vi "ImagerForFlowbit5_led_screenSensor.vi"() -> ()   [LabVIEW 2011]
uses:
  <vilib>/vision/Image Controls.llb/IMAQ Image.ctl
  <vilib>/Platform/TimedLoop/XDataNode/timing_clust.ctl
  <vilib>/Platform/TimedLoop/XDataNode/nitl_modes.ctl
  <vilib>/Platform/TimedLoop/XDataNode/wakeup.ctl
  <vilib>/Utility/config.llb/Read Key (I32).vi
  <vilib>/Analysis/1siggen.llb/Riffle Array (I32).vi
  <vilib>/Platform/TimedLoop/XDataNode/XDataNode.xnode
  <vilib>/Analysis/NI_AALBase.lvlib
  <vilib>/vision/NI_Vision_Development_Module.lvlib
  <vilib>/Platform/TimedLoop/XDataNode/XDNodeRunTimeDep.lvlib
  <vilib>/Utility/config.llb/NI_LVConfig.lvlib
panel:
  out "ScreenSensor":bool
  out "onLineMapOutput":T1[](array[typedef])
  out "Bounds.Right":i16
  out "停止循环":bool
  in  "Stimuli":i64=5
  in  "选项卡控件":enum32{"前面板", "参数设置", "OnLineMap"}(tab)
  in  "shutter":bool
  out "log":string
  out "Stim_ID":i32(listbox)=1
  in  "开始/暂停":bool=TRUE
  in  "停止":bool
  out "重排的 Stim ID":i32[](array[numeric]) caption="重排的{X}"
  out "block":i32
  out "队列中元素数量":i32
  out "Image 2":T1(plugin-control)
  in  "热图":bool
  out "循环持续时间":i64
  out "Recording":bool
  out "grabLoop":i32
  out "writeing data":bool
  out "address":i16=888 caption="地址" format="%.0x"
  in  "SaveParameter":bool
  in  "Pra_binType":enum16{"Extract", "Resample"}(ring)
  in  "Pra_FramesPerStim":i64=16
  in  "Pra_Blk目录":path=path "D:/Expt/test"
  in  "Pra_文件名":string="G4_E02"
  in  "Pra_TimeForPrepare(ms)":u32=1000
  in  "Pra_stim ID":u8[](array[numeric])=[0, 2, 4, 6, 8]
  in  "Pra_blk总数":i32=500
  in  "Pra_stim protocol":T2(array[ring])=[enum."prep stim", enum."wait respirator", enum."show stim", enum."recording data", enum."Blank stim", enum."writing data", enum."ISI"]
  in  "Pra_blank stim":u8
  in  "Pra_wait（ms）":u32=10
  in  "Pra_ISI（ms）":u32=8000
  in  "Pra_FrameBin":i32=25
  in  "Pra_datatype":u16(ring)=13 items=["U8"=11, "I16"=12, "U32"=13, "SGL"=14]
  in  "FrameWidth":i64=704
  in  "FrameHeight":i64=576
  in  "LoadParameter":bool
  in  "Pra_bin":enum16{"1*1", "2*2"}(ring)
  in  "Pra_DR/R parameter":T3={"frame_zero_0"=0, "frame_zero_1"=1, "frame_0"=3, "frame_1"=15}
  in  "Pra_OnlineMap":cluster{"数组 1":i32[], "数组 2":i32[]}[](array[cluster])=[{"数组 1"=[2], "数组 2"=[6]}, {"数组 1"=[4], "数组 2"=[8]}, {"数组 1"=[2, 6], "数组 2"=[4, 8]}, {"数组 1"=[2, 4, 6, 8], "数组 2"=[0]}, {"数组 1"=[2, 4], "数组 2"=[6, 8]}]
  in  "Pra_clip ratio":dbl=2.0 min=0.0001 step=0.1
  # "-"
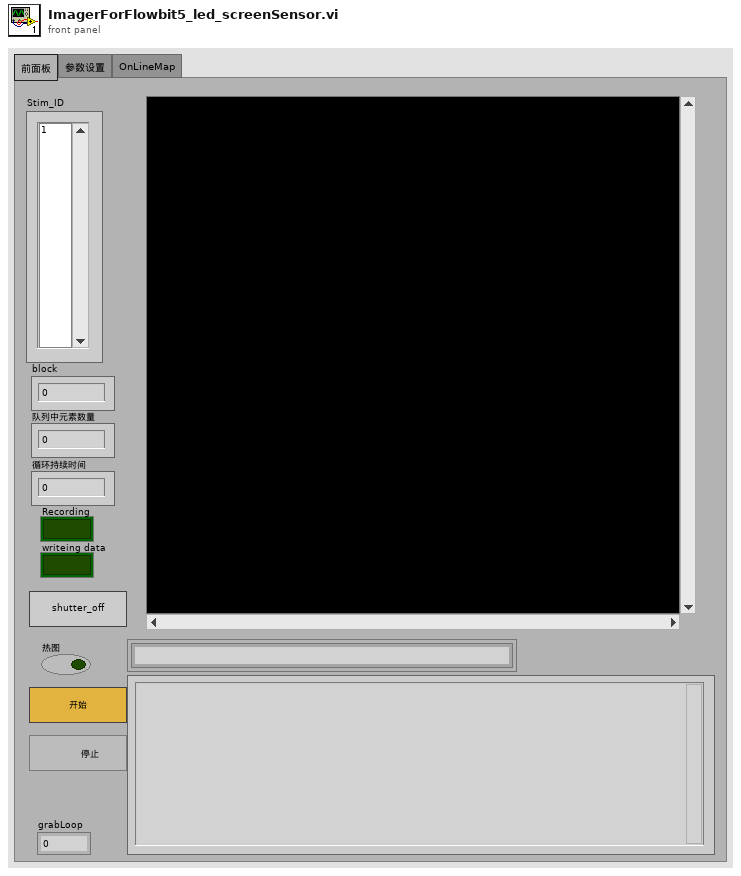
[diagram p1: front panel]
types:
  T1 = typedef "IMAQ Image.ctl" = refnum<image>
  T2 = enum16{"wait", "prep stim", "show stim", "wait respirator", "recording data", "Blank stim", "wait heart", "ISI", "DR/R", "wait calibrate", "openLightShutter", "closeLightShutter", "writing data"}[]
  T3 = cluster{"frame_zero_0":i32, "frame_zero_1":i32, "frame_0":i32, "frame_1":i32}
  T4 = typedef "Image Type" = u32
  T5 = enum16{"Disable External Trigger", "Enable External Trigger"}
  T6 = enum32{"Auto Detect", "RoadRunner", "Raven", "R64"}
  T7 = typedef "LVAllMonitorsDisplayTypeDef.ctl" = cluster{"Bounds":cluster{"Left":i16, "Top":i16, "Right":i16, "Bottom":i16}, "Depth":i16}[]
  T8 = cluster{"Bounds":cluster{"Left":i16, "Top":i16, "Right":i16, "Bottom":i16}, "Depth":i16}
  T9 = typedef "NI_LVConfig.lvlib/Config Data RefNum.ctl" = refnum<k1>
  T10 = typedef "XDNodeRunTimeDep.lvlib/timing_clust.ctl" = cluster{"Expected End [f-1]":u64, "Actual End [f-1]":u64, "Finished Late? [f-1]":bool, "Expected End [i-1]":u64, "Actual End [i-1]":u64, "Finished Late? [i-1]":bool, "Expected Start [i]":u64, "Actual Start [i]":u64, "Expected Start [f]":u64, "Actual Start [f]":u64, "Source Name":string, "Structure Name":string, "Period":i64, "Deadline":i64, "Offset":i64, "Start":i64, "Priority":i32, "Timeout":i32, "Mode":T11, "Wakeup Reason":T12, "Error":errorcluster, "Source Type":string, "Secondary Source Type":string, "Global End Time":u64, "Global Start Time":u64, "Frame Duration":u64, "Iteration Duration":u64, "Assigned CPU":i32, "I/O Scan Engine Mode":u32}
  T11 = typedef "XDNodeRunTimeDep.lvlib/nitl_modes.ctl" = enum32{"No Change", "Process missed periods, maintain original phase", "Discard missed periods, maintain original phase", "Process missed periods, ignore original phase", "Discard missed periods, ignore original phase"}
  T12 = typedef "XDNodeRunTimeDep.lvlib/wakeup.ctl" = enum32{"Normal", "Aborted", "Asynchronous wakeup", "Timing source error", "Timed loop error", "Timeout"}
  T13 = enum16{"big-endian, network order", "native, host order", "little-endian"}
  T14 = enum8{"Enabled", "Disabled", "Disabled and Grayed Out"}
  T15 = enum16{"open", "replace", "create", "open or create", "replace or create", "replace or create with confirmation"}
  T16 = cluster{"Browser Size":cluster{"X":i32, "Y":i32}, "Images per Line":i32, "Background Color":u32, "Frame Size":i32, "Frame Style":enum16{"Raised", "Bevelled", "Outline", "Hidden", "Step", "Raised Outline"}}
  T17 = cluster{"Desired Font (Application)":enum16{"User-specified Font", "Application Font", "System Font", "Dialog Font"}, "[User-specified Font]":cluster{"Font Name":string, "Size":i16, "Strikeout?":bool, "Italic?":bool, "Underline?":bool, "Outline?":bool, "Shadow?":bool, "Bold?":bool, "Rotation Angle":dbl}, "Horizontal Alignment":i16, "Vertical Alignment":i16}
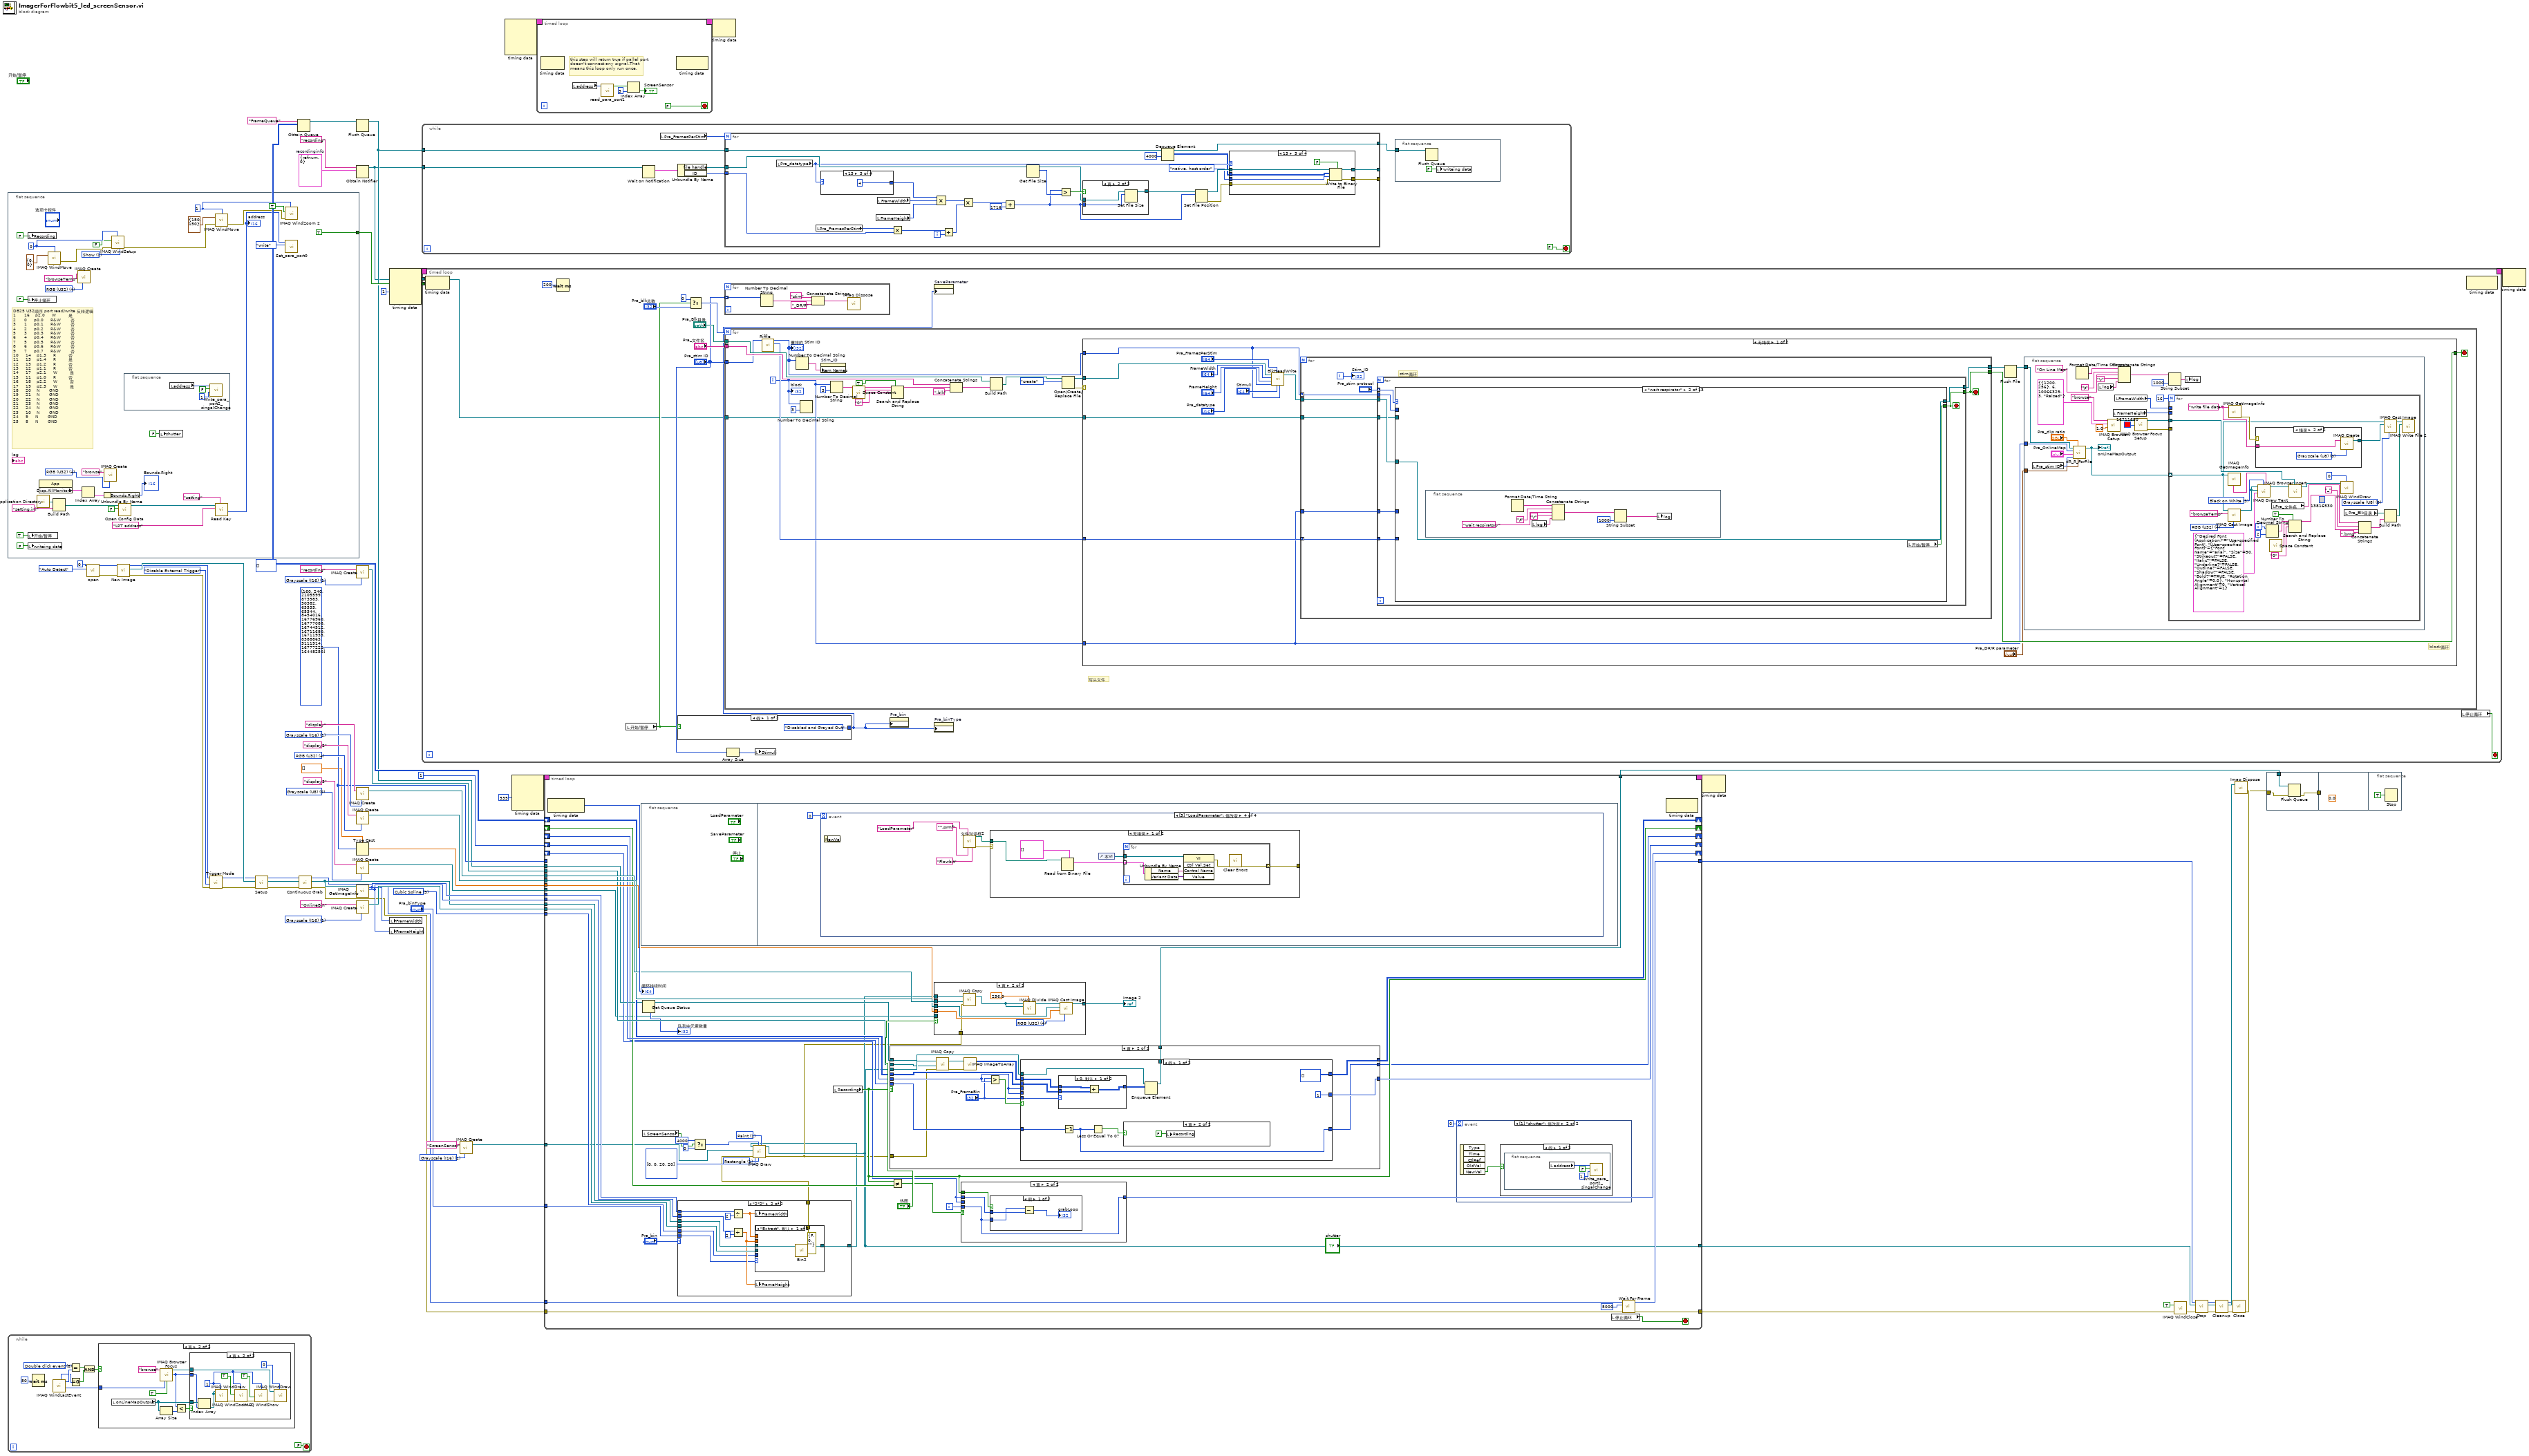
[diagram p0: block diagram]
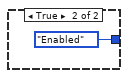
[diagram p2: hidden frame]
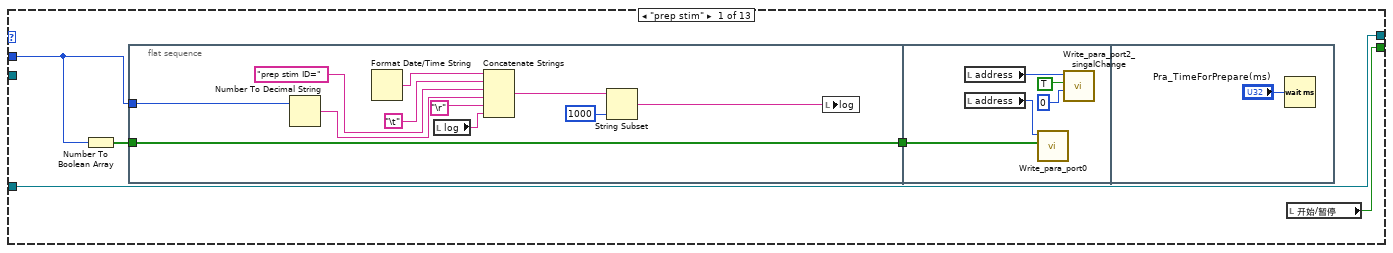
[diagram p4: hidden frame]
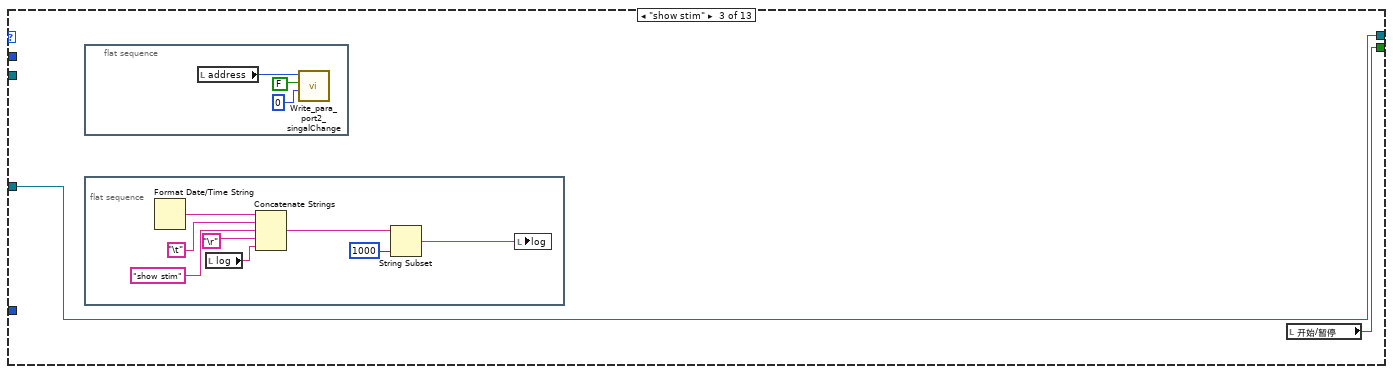
[diagram p5: hidden frame]
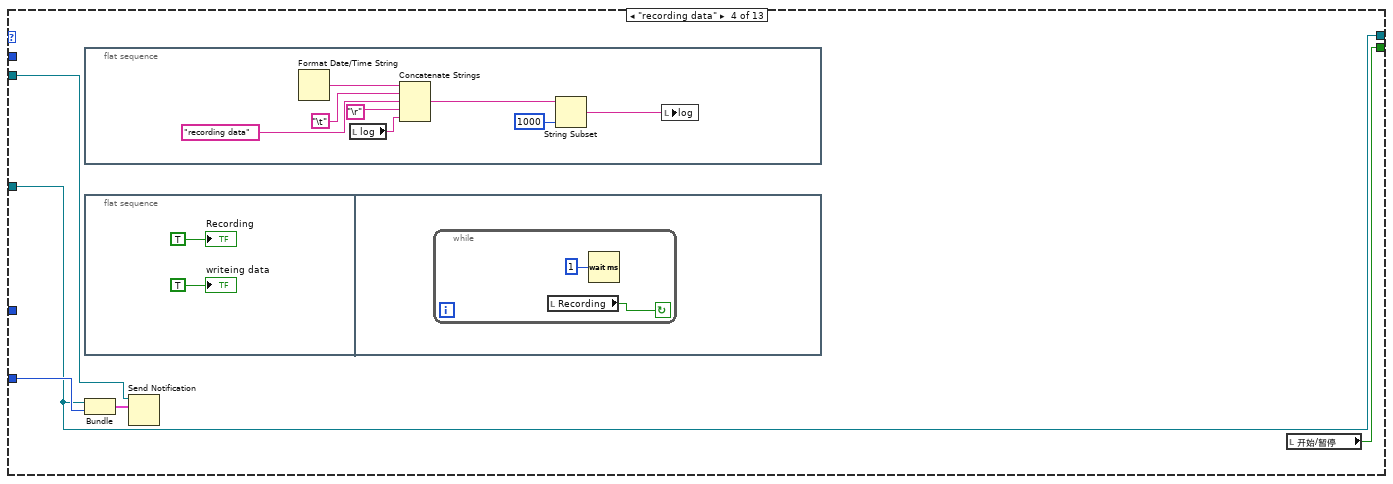
[diagram p6: hidden frame]
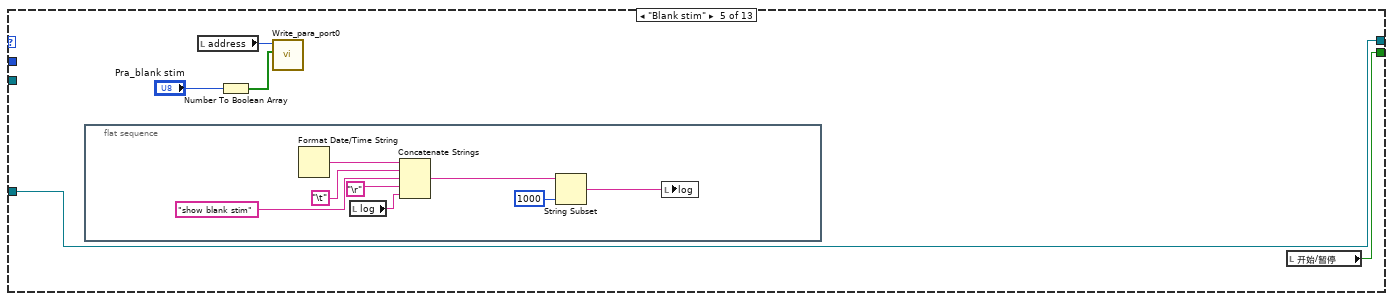
[diagram p7: hidden frame]
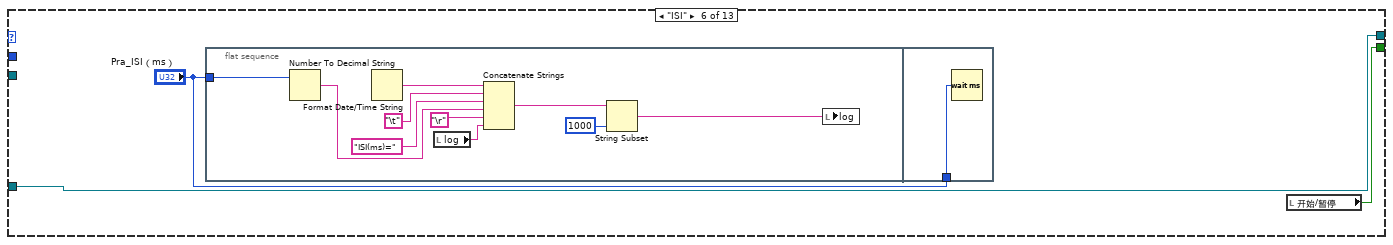
[diagram p8: hidden frame]
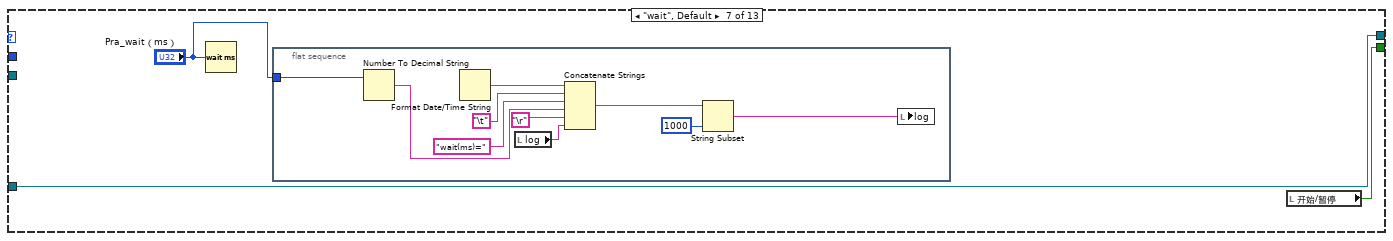
[diagram p9: hidden frame]
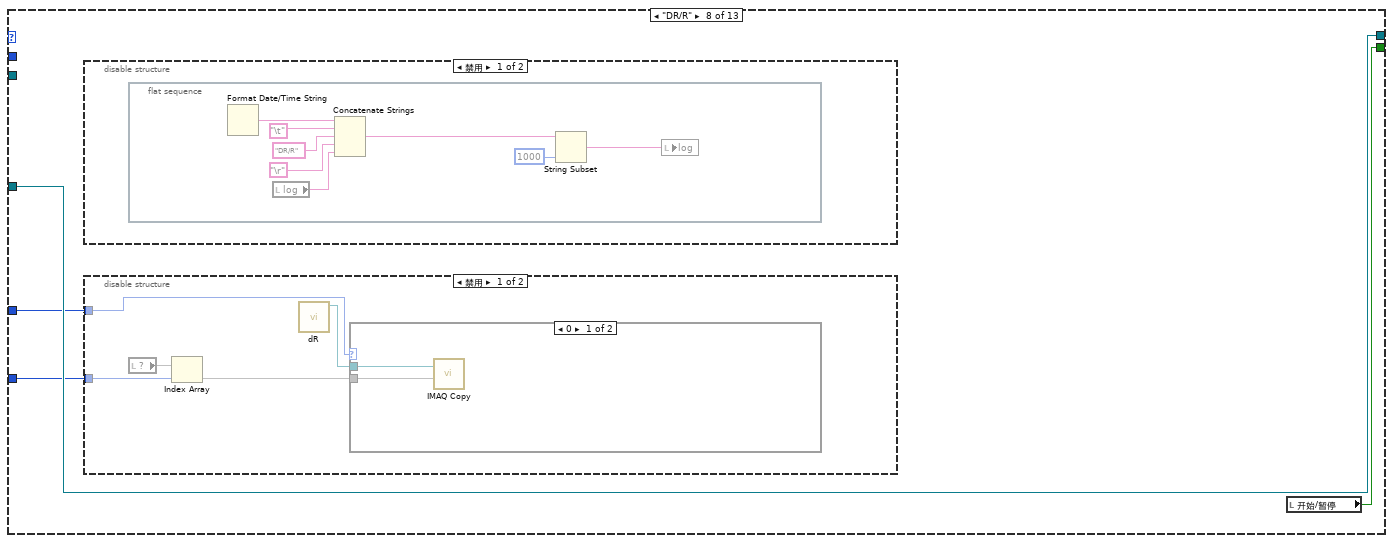
[diagram p10: hidden frame]
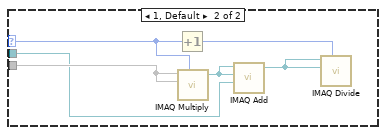
[diagram p12: hidden frame]
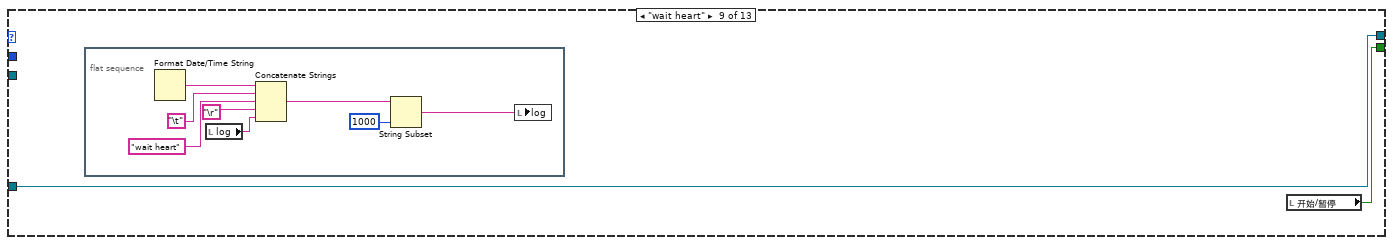
[diagram p14: hidden frame]
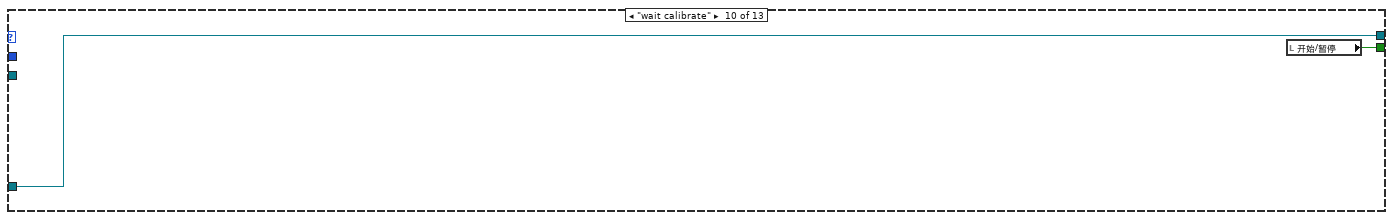
[diagram p15: hidden frame]
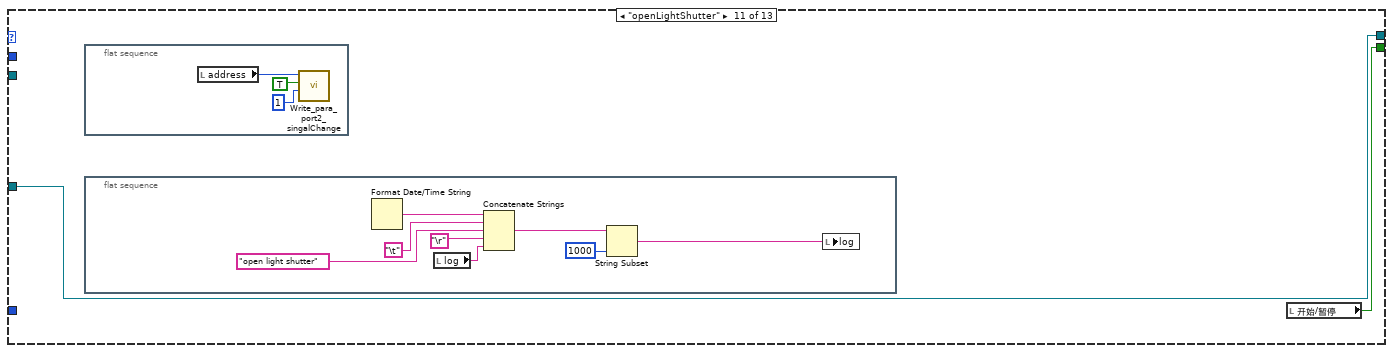
[diagram p16: hidden frame]
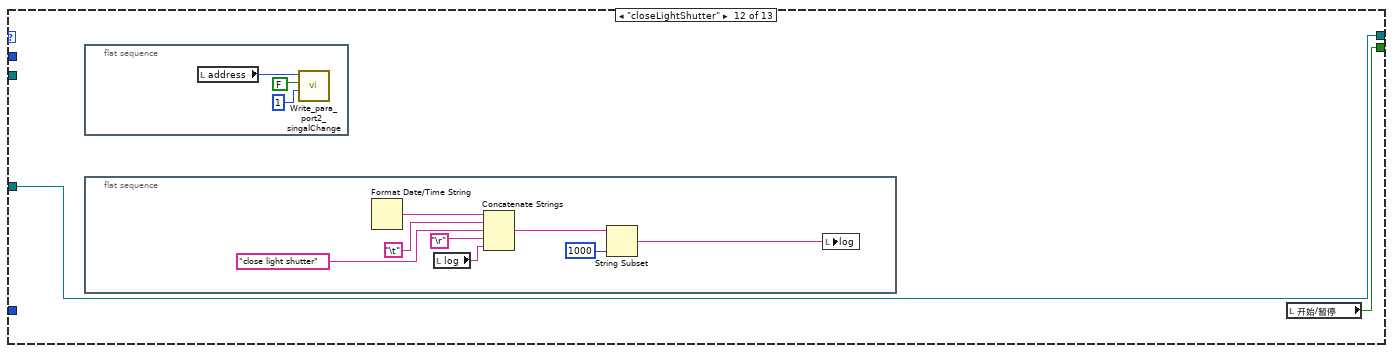
[diagram p17: hidden frame]
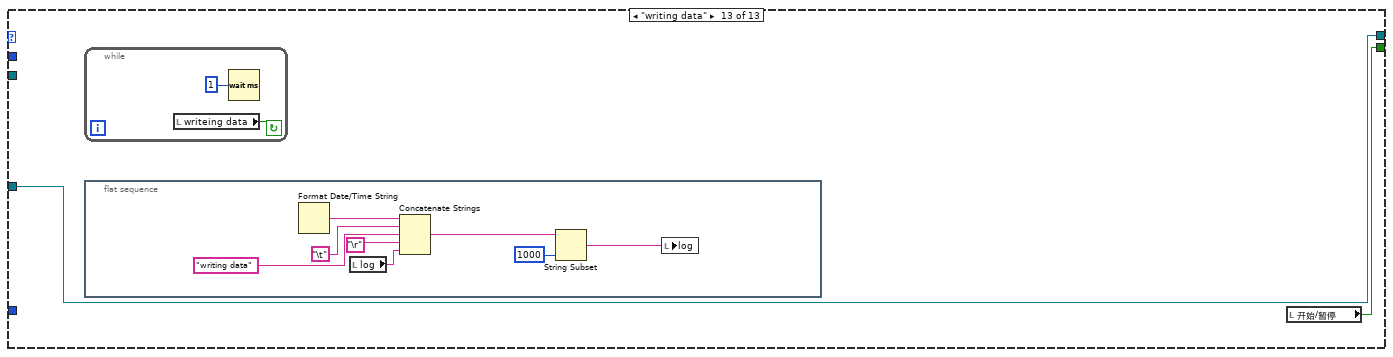
[diagram p18: hidden frame]
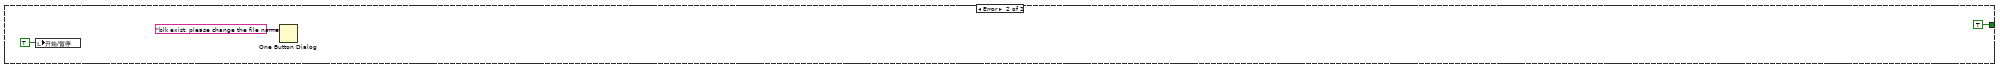
[diagram p19: hidden frame]
diagram:
  w6 = T4 1 items=["Grayscale (U8)", "Grayscale (I16)", "Grayscale (SGL)", "Complex (CSG)", "RGB (U32)", "HSL (U32)", "RGB (U64)", "Grayscale (U16)"] ("Image Type")
  w19 = cluster{"file handle":refnum<file>, "ID":i32} {"file handle"=refnum, "ID"=0}  # recordinginfo
  w24 = T4 0 items=["Grayscale (U8)", "Grayscale (I16)", "Grayscale (SGL)", "Complex (CSG)", "RGB (U32)", "HSL (U32)", "RGB (U64)", "Grayscale (U16)"] ("Image Type")
  w29 = u32 3 items=["Zero Order", "Bi-Linear", "Quadratic", "Cubic Spline"] ("Interpolation Type")
  w31 = T4 1 items=["Grayscale (U8)", "Grayscale (I16)", "Grayscale (SGL)", "Complex (CSG)", "RGB (U32)", "HSL (U32)", "RGB (U64)", "Grayscale (U16)"] ("Image Type")
  w33 = u32[][] []
  w42 = T4 4 items=["Grayscale (U8)", "Grayscale (I16)", "Grayscale (SGL)", "Complex (CSG)", "RGB (U32)", "HSL (U32)", "RGB (U64)", "Grayscale (U16)"] ("Image Type")
  w40 = u32[] [160, 240, 2105599, 873983, 50382, 65535, 65344, 8454016, 16776960, 16777088, 16744512, 16711680, 16711935, 8388863, 5111914, 16777222, 16448250] ("数组")
  w46 = T4 1 items=["Grayscale (U8)", "Grayscale (I16)", "Grayscale (SGL)", "Complex (CSG)", "RGB (U32)", "HSL (U32)", "RGB (U64)", "Grayscale (U16)"] ("Image Type")
  w47 = T4 1 items=["Grayscale (U8)", "Grayscale (I16)", "Grayscale (SGL)", "Complex (CSG)", "RGB (U32)", "HSL (U32)", "RGB (U64)", "Grayscale (U16)"] ("Image Type")
  n1 = flat-sequence {
    tunnel: [TRUE ("Zoom to Fit Mode")] -> w35
    frame #0 {
      w80 = 1 items=["Hide", "Show", "No change"] ("Scrollbars (No change)")
      w77 = 1 ("Window Number (0...15)")
      w81 = 0 ("Window Number (0...15)")
      w86 = T4 4 items=["Grayscale (U8)", "Grayscale (I16)", "Grayscale (SGL)", "Complex (CSG)", "RGB (U32)", "HSL (U32)", "RGB (U64)", "Grayscale (U16)"] ("Image Type")
      w87 = T4 4 items=["Grayscale (U8)", "Grayscale (I16)", "Grayscale (SGL)", "Complex (CSG)", "RGB (U32)", "HSL (U32)", "RGB (U64)", "Grayscale (U16)"] ("Image Type")
      # "DB25\tU32顺序\tport\tread/write\t反转逻辑\n1\t     16\t   p2.0    \tW\t        是\n2\t     0    \tp0.0\t   \tR&W\t      否\n3\t     1\t\t   p0.1\t   \tR&W      \t否\n4\t\t    2\t   \tp0.2   \t\tR&W      \t否\n5\t\t    3\t\t   p0.3   \t\tR&W\t      否\n6\t\t    4\t   \tp0.4   \t\tR&W      \t否\n7\t\t    5\t   \tp0.5   \t\tR&W      \t否\n8\t\t    6\t   \tp0.6\t   \tR&W      \t否\n9\t    \t7\t   \tp0.7\t   \tR&W\t      否\n10\t    14   \tp1.3   \t\tR        \t否\n11\t   \t15   \tp1.4   \t\tR        \t是\n12\t   \t13   \tp1.2\t   \tR        \t否\n13    \t12   \tp1.1\t   \tR        \t否\n14     17   \tp2.1\t   \tW        \t是\n15    \t11   \tp1.0   \t\tR\t        否\n16    \t18   \tp2.2   \t\tW        \t否\n17    \t19\t   p2.3   \t\tW\t        是\n18    \t20   \tN   \t  \tGND\t\n19    \t21   \tN   \t  \tGND\t\n20\t    22\t   N\t  \t  \tGND\t\n21\t    23\t   N  \t  \t\tGND\t\n22\t    24\t   N  \t  \t\tGND\t\n23    \t10   \tN  \t  \t\tGND\t\n24    \t9\t    N  \t  \t\tGND\t\n25\t    8    \tN  \t  \t\tGND"
      n2 = local write "Recording"(FALSE ("Recording")) -> ()
      n3 = local write "停止循环"(FALSE ("开始/暂停")) -> ()
      n4 = local write "开始/暂停"(TRUE ("开始/暂停")) -> ()
      n5 = local write "writeing data"(FALSE ("Recording")) -> ()
      n6 = call <vilib>:"Application Directory.vi"() -> ("Application Directory"=w99:path)
      n7 = property class="App"() -> ("Disp.AllMonitors"=w91:T7)  [unwired: 2 in, 2 out]
      n8 = call "IMAQ WindMove"("Window Number (0...15)"=w81, "Coordinates (screen)"=cluster{"X Position":i32, "Y Position":i32} {"X Position"=0, "Y Position"=0}) -> ("error out"=w82:errorcluster)  [unwired: 3 in, 1 out]
      n9 = Build Path(base path=w99, name or relative path="setting.ini" ("名称或相对路径")) -> (appended path=w97:path)
      n10 = call "IMAQ Create"("Image Name"="browseTemp", "Image Type"=w86) -> ()  [unwired: 3 in, 2 out]
      n11 = Index Array(array=w91) -> (element=w90:T8)  [unwired: 1 in]
      n12 = call "IMAQ Create"("Image Name"="browse", "Image Type"=w87) -> ()  [unwired: 3 in, 2 out]
      n13 = Unbundle By Name(w90) -> ("Bounds.Right"=→"Bounds.Right":i16)
      n14 = call "IMAQ WindSetup"("Scrollbars (No change)"=w80, "Window Number (0...15)"=w81, "error in (no error)"=w82, "Window can close? (Yes)"=FALSE) -> ("error out"=w79:errorcluster)  [unwired: 7 in]
      n15 = call <vilib>:"Open Config Data.vi"("create file if necessary (T)"=FALSE, "configuration file path"=w97) -> ("refnum"=w95:T9)  [unwired: 7 in, 2 out]
      n16 = flat-sequence {
        frame #0 {
          n17 = local read "address"() -> (w106:i16)
          n18 = call "Write_para_port2_singalChange.vi"("索引"=1, "布尔"=FALSE, "address"=w106) -> ()  [unwired: 8 in, 1 out]
        }
      }
      n19 = local write "shutter"(FALSE ("shutter")) -> ()
      n20 = call "IMAQ WindMove"("Window Number (0...15)"=w77, "Coordinates (screen)"=cluster{"X Position":i32, "Y Position":i32} {"X Position"=150, "Y Position"=150}, "error in (no error)"=w79) -> ("error out"=w78:errorcluster)  [unwired: 2 in, 1 out]
      n21 = call-poly <vilib>:"Read Key.vi"("section"="setting", "key"="LPT address", "refnum"=w95) -> ("value"=w92:i32)  [unwired: 5 in, 3 out]
      "address" <- w92
      n22 = call "IMAQ WindZoom 2"("Window Number (0...15)"=w77, "error in (no error)"=w78, "Zoom to Fit? (False)"=TRUE) -> ()  [unwired: 5 in, 4 out]
      n23 = call "Set_para_port0.vi"("R or W"=enum16{"read", "write"}."write", "address"=w92) -> ()  [unwired: 8 in, 2 out]
    }
  }
  n24 = while {
    stop <- FALSE stop-if-true
    w115 = 8 items=["No  event", "Click event", "Draw event", "Move event", "Size event", "Scroll event", "Activate event", "Close event", "Double click event"] ("Event")
    n25 = Wait (ms)(milliseconds to wait=u32 50 ("等待时间（毫秒）")) -> ()  [unwired: 1 out]
    n26 = call "IMAQ WindLastEvent"() -> ("Coordinates"=w109:i32[], "Event"=w114:i32, "Window Number (0...15)"=w113:i32)  [unwired: 6 in, 3 out]
    n27 = Equal?(x=w115, y=w114) -> (x = y?=w112:bool)
    n28 = Equal To 0?(x=w113) -> (x = 0?=w111:bool)
    n29 = And(x=w112, y=w111) -> (x .and. y?=w110:bool)
    n30 = case shown="真" w110 {
      tunnel: w109 -> [_ w125]
      frame False {
      }
      frame True {
        n31 = local read "onLineMapOutput"() -> (w121:T1[])
        n32 = call "IMAQ Browser Focus"("Image Browser In"="browse" ("Image Name"), "Pixel Position"=w125, "Get/Set (Set)"=TRUE) -> ("Image Browser Out"=w119:T1, "Index Out"=w120:i32)  [unwired: 5 in, 6 out]
        n33 = Array Size(array=w121) -> (size(s)=w123:i32)
        n34 = Less?(x=w120, y=w123) -> (x < y?=w122:bool)
        n35 = case shown="真" w122 {
          tunnel: w121 -> [_ w136]
          tunnel: w120 -> [_ w135]
          tunnel: w119 -> [_ w133]
          frame False {
          }
          frame True {
            w127 = 1 ("Window Number (0...15)")
            n36 = Index Array(array=w136, index=w135) -> (element=w134:T1)
            n37 = call "IMAQ WindDraw"("Window Number (0...15)"=w127, "Title"=w134, "Image"=w134) -> ("error out"=w130:errorcluster)  [unwired: 7 in, 1 out]
            n38 = call "IMAQ WindZoom 2"("Window Number (0...15)"=w127, "error in (no error)"=w130, "Zoom to Fit? (False)"=TRUE) -> ("error out"=w129:errorcluster)  [unwired: 5 in, 3 out]
            n39 = call "IMAQ WindShow"("error in (no error)"=w129, "Bring To Front? (N)"=TRUE, "Window Number (0...15)"=w127) -> ("error out"=w128:errorcluster)  [unwired: 3 in, 2 out]
            n40 = call "IMAQ WindDraw"("Window Number (0...15)"=0, "error in (no error)"=w128, "Image"=w133) -> ()  [unwired: 7 in, 2 out]
          }
        }
      }
    }
  }
  n41 = call <vilib>:"open.vi"("Board Type"=T6."Auto Detect", "Board Number"=u32 0) -> ("error out"=w61:errorcluster, "RefBrdOut"=w57:u32)  [unwired: 2 in, 5 out]
  n42 = call <vilib>:"New Image.vi"("RefBrdIn"=w57, "error in"=w61) -> ("RefBrdOut"=w56:u32, "Image"=w69:T1, "error out"=w62:errorcluster)  [unwired: 6 in]
  n43 = call <vilib>:"Trigger Mode.vi"("RefBrdIn"=w56, "Trigger Mode"=T5."Disable External Trigger", "error in (no error)"=w62) -> ("RefBrdOut"=w55:u32, "error out"=w63:errorcluster)  [unwired: 6 in]
  n44 = call <vilib>:"Setup.vi"("error in"=w63, "Image In"=w69, "RefBrdIn"=w55) -> ("error out"=w58:errorcluster, "Image"=w59:T1, "RefBrdOut"=w54:u32)  [unwired: 6 in]
  n45 = Obtain Queue(name (unnamed)="FrameQueue" ("名称（未命名）"), element data type=w33) -> (queue out=w36:refnum<queue>)  [unwired: 3 in, 2 out]
  n46 = call <vilib>:"Continuous Grab.vi"("error in (no error)"=w58, "Image In"=w59, "RefBrdIn"=w54) -> ("error out"=w13:errorcluster, "Image"=w25:T1, "RefBrdOut"=w14:u32)  [unwired: 6 in]
  n47 = Flush Queue(queue=w36) -> (queue out=w21:refnum<queue>)  [unwired: 1 in, 2 out]
  n48 = Obtain Notifier(name (unnamed)="recording" ("名称（未命名）"), notification data type=w19) -> (notifier out=w18:refnum<notifier>)  [unwired: 2 in, 2 out]
  n49 = call "IMAQ Create"("Image Name"="recording", "Image Type"=w47) -> ("New Image"=w49:T1)  [unwired: 3 in, 1 out]
  n50 = call "IMAQ Create"("Image Name"="display", "Image Type"=w46) -> ("New Image"=w44:T1)  [unwired: 3 in, 1 out]
  n51 = call "IMAQ Create"("Image Name"="display2", "Image Type"=w42) -> ("New Image"=w41:T1)  [unwired: 3 in, 1 out]
  n52 = Type Cast(type=sgl[] [] ("单精度浮点"), x=w40) -> (*(type *) &x=w38:sgl[])
  n53 = call "IMAQ Create"("Image Name"="display3", "Image Type"=w24) -> ("New Image"=w22:T1)  [unwired: 3 in, 1 out]
  n54 = call "IMAQ GetImageInfo"("Image"=w25) -> ("Y Resolution"=w27:i32, "X Resolution"=w28:i32)  [unwired: 3 in, 6 out]
  n55 = call "IMAQ Create"("Image Name"="OnlineBin", "Image Type"=w31) -> ("New Image"=w30:T1)  [unwired: 3 in, 1 out]
  n56 = node-c288(1 ("优先级")) -> (w4:T10)  [unwired: 3 in]
  n57 = local write "FrameWidth"(w28) -> ()
  n58 = local write "FrameHeight"(w27) -> ()
  n59 = while {
    tunnel: w21 -> [w143]
    tunnel: w18 -> [w141]
    stop <- FALSE stop-if-true
    n60 = Wait on Notification(notifier=w141) -> (notification=w140:cluster{"file handle":refnum<file>, "ID":i32})  [unwired: 3 in, 3 out]
    n61 = local read "Pra_FramesPerStim"() -> (w142:i64)
    n62 = Unbundle By Name(w140) -> ("file handle"=w139:refnum<file>, "ID"=w138:i32)
    n63 = for {
      N: w142 -> [_]
      tunnel: w139 -> [w173]
      tunnel: w138 -> [w157]
      tunnel: [w165] -> _
      tunnel: [w164] -> w137
      tunnel: w143 -> [w149]
      tunnel: [w147] -> _
      i -> [w155]
      n64 = local read "Pra_datatype"() -> (w169:u16)
      n65 = local read "Pra_FramesPerStim"() -> (w158:i64)
      n66 = case shown="13" w169 {
        tunnel: [i64 1 i64 2 i64 4 i64 4] -> w161
        frame 11, Default {
        }
        frame 12 {
        }
        frame 13 {
        }
        frame 14 {
        }
      }
      n67 = local read "FrameHeight"() -> (w159:i64)
      n68 = local read "FrameWidth"() -> (w160:i64)
      n69 = Multiply(x=w158, y=w157) -> (x*y=w156:i64)
      n70 = Compound Arithmetic op=MULTIPLY(w161, w160, w159) -> (w153:i64)
      n71 = Add(x=w156, y=w155) -> (x+y=w154:i64)
      n72 = Multiply(x=w153, y=w154) -> (x*y=w152:i64)
      n73 = Add(x=w152, y=i64 1716 ("x")) -> (x+y=w150:i64)
      n74 = Get File Size(file=w173) -> (refnum out=w166:refnum<file>, size (in bytes)=w162:i64)  [unwired: 1 in, 1 out]
      n75 = Greater?(x=w150, y=w162) -> (0:w167:bool)
      n76 = case shown="真" w167 {
        tunnel: w150 -> [_ w208]
        tunnel: w166 -> [w205 w207]
        tunnel: [w205 w206] -> w168
        frame False {
        }
        frame True {
          n77 = Set File Size(6:w208, 7:w207) -> (3:w206:refnum<file>)  [unwired: 1 in, 1 out]
        }
      }
      n78 = Dequeue Element(queue=w149, timeout in ms (-1)=4000 ("超时毫秒(-1)")) -> (queue out=w164:refnum<queue>, element=w148:u32[][])  [unwired: 1 in, 2 out]
      n79 = Set File Position(offset (in bytes) (0)=w150, refnum=w168) -> (refnum out=w172:refnum<file>, error out=w170:errorcluster)  [unwired: 2 in]
      n80 = case shown="13" w169 {
        tunnel: w148 -> [w176 w185 w191 w198]
        tunnel: w172 -> [w180 w186 w194 w200]
        tunnel: T13."native, host order" ("字节顺序(0:big-endian, network order)") -> [w179 w187 w192 w201]
        tunnel: w170 -> [w178 w182 w193 w202]
        tunnel: [w177 w188 w195 w203] -> w165
        tunnel: [w174 w183 w190 w197] -> w147
        frame 11, Default {
          n81 = To Unsigned Byte Integer(number=w176) -> (unsigned 8bit integer=w175:u8[][])
          n82 = Write to Binary File(file (use dialog)=w180, data=w175, error in=w178, 5:FALSE ("预置数组或字符串大小？(T)"), 9:w179) -> (refnum out=w177:refnum<file>, error out=w174:errorcluster)  [unwired: 1 in, 1 out]
        }
        frame 12 {
          n83 = To Unsigned Word Integer(number=w185) -> (unsigned 16bit integer=w184:u16[][])
          n84 = Write to Binary File(file (use dialog)=w186, data=w184, error in=w182, 5:FALSE ("预置数组或字符串大小？(T)"), 9:w187) -> (refnum out=w188:refnum<file>, error out=w183:errorcluster)  [unwired: 1 in, 1 out]
        }
        frame 13 {
          n85 = Write to Binary File(file (use dialog)=w194, data=w191, error in=w193, 5:FALSE ("预置数组或字符串大小？(T)"), 9:w192) -> (refnum out=w195:refnum<file>, error out=w190:errorcluster)  [unwired: 1 in, 1 out]
        }
        frame 14 {
          n86 = To Single Precision Float(number=w198) -> (single precision float=w199:sgl[][])
          n87 = Write to Binary File(file (use dialog)=w200, data=w199, error in=w202, 5:FALSE ("预置数组或字符串大小？(T)"), 9:w201) -> (refnum out=w203:refnum<file>, error out=w197:errorcluster)  [unwired: 1 in, 1 out]
        }
      }
    }
    n88 = flat-sequence {
      tunnel: w137 -> [w146]
      frame #0 {
        n89 = Flush Queue(queue=w146) -> ()  [unwired: 1 in, 3 out]
        n90 = local write "writeing data"(FALSE ("writeing data")) -> ()
      }
    }
  }
  n91 = timed-loop {
    tunnel: w35 -> [_]
    tunnel: w18 -> [w213]
    timing: w4 -> [_]
    timing-out: [_] -> w3
    stop <- w223 stop-if-true
    n92 = node-c288() -> ()  [unwired: 1 in, 1 out]
    n93 = Wait (ms)(milliseconds to wait=u32 200 ("等待时间（毫秒）")) -> ()  [unwired: 1 out]
    n94 = local read "开始/暂停"() -> (w215:bool)
    n95 = case shown="假" w215 {
      tunnel: [T14."Disabled and Grayed Out" ("禁用") T14."Enabled" ("禁用")] -> w214
      frame False {
      }
      frame True {
      }
    }
    n96 = Select(t=0, s=w215, f="Pra_blk总数") -> (s? t:f=w220:i32)
    n97 = for {
      tunnel: "Pra_stim ID" -> [w230] mode=indexing
      n98 = Number To Decimal String(number=w230) -> (decimal integer string=w231:string)  [unwired: 1 in]
      n99 = Concatenate Strings("stim" ("字符串"), w231, "_DR/R" ("字符串")) -> (w229:string)
      n100 = call "Imaq Dispose"("Image"=w229) -> ()  [unwired: 5 in, 1 out]
    }
    n101 = for {
      N: w220 -> [_]
      tunnel: "Pra_stim ID" -> [w251]
      tunnel: "Pra_文件名" -> [w255]
      tunnel: "Pra_Blk目录" -> [w254]
      tunnel: w213 -> [w247]
      i -> [w249]
      stop <- w252 stop-if-true
      # "写头文件"
      n102 = call-poly <vilib>:"Riffle.vi"("X"=w251) -> ("Riffled Index"=w250:i32[], "Riffled {X}"=w253:i32[])  [unwired: 8 in, 1 out]
      "重排的 Stim ID" <- w253
      n103 = Number To Decimal String(number=w253) -> (decimal integer string=w237:string[])  [unwired: 1 in]
      n104 = Number To Decimal String(number=w249, width (-)=i16 3 ("宽度(-)")) -> ()  [unwired: 1 out]
      n105 = property on="Stim_ID" class="LstBox (严格)"("Item Names"=w237) -> ()  [unwired: 2 in, 2 out]
      n106 = Number To Decimal String(number=w249, width (-)=i16 3 ("宽度(-)")) -> (decimal integer string=w242:string)
      n107 = call <vilib>:"Space Constant.vi"() -> ("String"=w243:string)
      n108 = Search and Replace String(replace all?=TRUE ("替换全部？(F)"), input string=w242, search string=w243, replace string="0" ("替换字符串(\"\")")) -> (result string=w240:string)  [unwired: 4 in, 3 out]
      n109 = Concatenate Strings(w255, w240, ".blk" ("字符串")) -> (w238:string)
      n110 = Build Path(base path=w254, name or relative path=w238) -> (appended path=w248:path)
      n111 = Open/Create/Replace File(file path (use dialog)=w248, operation (0:open)=T15."create" ("操作(0:open)")) -> (refnum out=w235:refnum<file>, error out=w234:errorcluster)  [unwired: 4 in, 1 out]
      n112 = case shown="无错误" w234 {
        tunnel: w253 -> [w256 _]
        tunnel: [w269 TRUE ("开始/暂停")] -> w252
        tunnel: w250 -> [w268 _]
        tunnel: w249 -> [w266 _]
        tunnel: w247 -> [w263 _]
        tunnel: w235 -> [w258 _]
        frame No Error {
          # "block循环"
          n113 = call "BlkHeadWrite.vi"("SequenceOfID"=w256, "Stimuli"="Stimuli", "FramesPerStim"="Pra_FramesPerStim", "datatype"="Pra_datatype", "FrameHeight"="FrameHeight", "FrameWidth"="FrameWidth", "引用句柄输入"=w258) -> ("引用句柄输出"=w270:refnum<file>)  [unwired: 4 in]
          n114 = for {
            tunnel: w270 -> [w337]
            tunnel: [w335] -> w265
            tunnel: w268 -> [w336] mode=indexing
            tunnel: w256 -> [w334] mode=indexing
            tunnel: [w333] -> w269
            tunnel: w266 -> [w330]
            tunnel: w263 -> [w329]
            i -> [w332]
            stop <- w333 stop-if-true
            # "stim循环"
            n115 = for {
              tunnel: w336 -> [w344]
              tunnel: w334 -> [w342]
              tunnel: [w340] -> w333
              tunnel: "Pra_stim protocol" -> [w341] mode=indexing
              tunnel: w337 -> [w345]
              tunnel: [w343] -> w335
              tunnel: w330 -> [w339]
              tunnel: w329 -> [w338]
              stop <- w340 stop-if-true
              n116 = case shown="\"wait respirator\"" w341 {
                tunnel: w345 -> [w348 w368 w378 w392 w409 w422 w436 w451 w473 w483 w485 w498 w511]
                tunnel: w344 -> [_ _ _ w394 _ _ _ w449 _ _ _ _ _]
                tunnel: [w348 w368 w378 w392 w409 w422 w436 w451 w473 w483 w485 w498 w511] -> w343
                tunnel: w342 -> [w346 _ _ _ _ _ _ _ _ _ _ _ _]
                tunnel: [w349 w369 w379 w391 w410 w423 w437 w450 w474 w484 w486 w499 w512] -> w340
                tunnel: w339 -> [_ _ _ _ _ _ _ w448 _ _ _ _ _]
                tunnel: w338 -> [_ _ _ w395 _ _ _ _ _ _ _ _ _]
                frame "prep stim" {
                  n117 = Number To Boolean Array(number=w346) -> (Boolean array=w350:bool[])
                  n118 = flat-sequence {
                    tunnel: w350 -> [w361]
                    tunnel: [w361] -> w347
                    tunnel: w346 -> [w360]
                    tunnel: w347 -> [w366]
                    frame #0 {
                      n119 = Number To Decimal String(number=w360) -> (decimal integer string=w357:string)  [unwired: 1 in]
                      n120 = Format Date/Time String() -> (date/time string=w359:string)  [unwired: 3 in]
                      n121 = local read "log"() -> (w353:string)
                      n122 = Concatenate Strings(w359, "\t", "prep stim ID=" ("字符串"), w357, "\r", w353) -> (w355:string)
                      n123 = String Subset(string=w355, length (rest)=1000 ("y")) -> (substring=w354:string)  [unwired: 1 in]
                      n124 = local write "log"(w354) -> ()
                    }
                    frame #1 {
                      n125 = local read "address"() -> (w363:i16)
                      n126 = local read "address"() -> (w362:i16)
                      n127 = call "Write_para_port0.vi"("port0（8元素）"=w366, "address"=w362) -> ()  [unwired: 9 in, 1 out]
                      n128 = call "Write_para_port2_singalChange.vi"("索引"=0, "布尔"=TRUE, "address"=w363) -> ()  [unwired: 8 in, 1 out]
                    }
                    frame #2 {
                      n129 = Wait (ms)(milliseconds to wait="Pra_TimeForPrepare(ms)") -> ()  [unwired: 1 out]
                    }
                  }
                  n130 = local read "开始/暂停"() -> (w349:bool)
                }
                frame "wait respirator" {
                  n131 = flat-sequence {
                    frame #0 {
                      n132 = Format Date/Time String() -> (date/time string=w377:string)  [unwired: 3 in]
                      n133 = local read "log"() -> (w372:string)
                      n134 = Concatenate Strings(w377, "\t", "wait respiratory" ("字符串"), "\r", w372) -> (w374:string)
                      n135 = String Subset(string=w374, length (rest)=1000 ("y")) -> (substring=w373:string)  [unwired: 1 in]
                      n136 = local write "log"(w373) -> ()
                    }
                  }
                  n137 = local read "开始/暂停"() -> (w369:bool)
                }
                frame "show stim" {
                  n138 = flat-sequence {
                    frame #0 {
                      n139 = local read "address"() -> (w388:i16)
                      n140 = call "Write_para_port2_singalChange.vi"("索引"=0, "布尔"=FALSE, "address"=w388) -> ()  [unwired: 8 in, 1 out]
                    }
                  }
                  n141 = flat-sequence {
                    frame #0 {
                      n142 = Format Date/Time String() -> (date/time string=w387:string)  [unwired: 3 in]
                      n143 = local read "log"() -> (w382:string)
                      n144 = Concatenate Strings(w387, "\t", "show stim" ("字符串"), "\r", w382) -> (w384:string)
                      n145 = String Subset(string=w384, length (rest)=1000 ("y")) -> (substring=w383:string)  [unwired: 1 in]
                      n146 = local write "log"(w383) -> ()
                    }
                  }
                  n147 = local read "开始/暂停"() -> (w379:bool)
                }
                frame "recording data" {
                  n148 = flat-sequence {
                    frame #0 {
                      n149 = Format Date/Time String() -> (date/time string=w407:string)  [unwired: 3 in]
                      n150 = local read "log"() -> (w402:string)
                      n151 = Concatenate Strings(w407, "\t", "recording data" ("字符串"), "\r", w402) -> (w404:string)
                      n152 = String Subset(string=w404, length (rest)=1000 ("y")) -> (substring=w403:string)  [unwired: 1 in]
                      n153 = local write "log"(w403) -> ()
                    }
                  }
                  n154 = flat-sequence {
                    frame #0 {
                      "Recording" <- TRUE ("Recording")
                      "writeing data" <- TRUE ("Recording")
                    }
                    frame #1 {
                      n155 = while {
                        stop <- w399 continue-if-true
                        n156 = local read "Recording"() -> (w399:bool)
                        n157 = Wait (ms)(milliseconds to wait=u32 1 ("等待时间（毫秒）")) -> ()  [unwired: 1 out]
                      }
                    }
                  }
                  n158 = Bundle("引用句柄输出"=w392, w394) -> (w393:cluster{"引用句柄输出":refnum<file>, i32})  [unwired: 1 in]
                  n159 = Send Notification(notification=w393, notifier=w395) -> ()  [unwired: 1 in, 2 out]
                  n160 = local read "开始/暂停"() -> (w391:bool)
                }
                frame "Blank stim" {
                  n161 = flat-sequence {
                    frame #0 {
                      n162 = Format Date/Time String() -> (date/time string=w420:string)  [unwired: 3 in]
                      n163 = local read "log"() -> (w415:string)
                      n164 = Concatenate Strings(w420, "\t", "show blank stim" ("字符串"), "\r", w415) -> (w417:string)
                      n165 = String Subset(string=w417, length (rest)=1000 ("y")) -> (substring=w416:string)  [unwired: 1 in]
                      n166 = local write "log"(w416) -> ()
                    }
                  }
                  n167 = local read "address"() -> (w408:i16)
                  n168 = Number To Boolean Array(number="Pra_blank stim") -> (Boolean array=w411:bool[])
                  n169 = call "Write_para_port0.vi"("port0（8元素）"=w411, "address"=w408) -> ()  [unwired: 9 in, 1 out]
                  n170 = local read "开始/暂停"() -> (w410:bool)
                }
                frame "ISI" {
                  n171 = flat-sequence {
                    tunnel: "Pra_ISI（ms）" -> [w427]
                    tunnel: "Pra_ISI（ms）" -> [w434]
                    frame #0 {
                      n172 = Number To Decimal String(number=w427) -> (decimal integer string=w431:string)  [unwired: 1 in]
                      n173 = Format Date/Time String() -> (date/time string=w433:string)  [unwired: 3 in]
                      n174 = local read "log"() -> (w426:string)
                      n175 = Concatenate Strings(w433, "\t", "ISI(ms)=" ("字符串"), w431, "\r", w426) -> (w429:string)
                      n176 = String Subset(string=w429, length (rest)=1000 ("y")) -> (substring=w428:string)  [unwired: 1 in]
                      n177 = local write "log"(w428) -> ()
                    }
                    frame #1 {
                      n178 = Wait (ms)(milliseconds to wait=w434) -> ()  [unwired: 1 out]
                    }
                  }
                  n179 = local read "开始/暂停"() -> (w423:bool)
                }
                frame "wait", Default {
                  n180 = Wait (ms)(milliseconds to wait="Pra_wait（ms）") -> ()  [unwired: 1 out]
                  n181 = flat-sequence {
                    tunnel: "Pra_wait（ms）" -> [w441]
                    frame #0 {
                      n182 = Number To Decimal String(number=w441) -> (decimal integer string=w445:string)  [unwired: 1 in]
                      n183 = Format Date/Time String() -> (date/time string=w447:string)  [unwired: 3 in]
                      n184 = local read "log"() -> (w440:string)
                      n185 = Concatenate Strings(w447, "\t", "wait(ms)=" ("字符串"), w445, "\r", w440) -> (w443:string)
                      n186 = String Subset(string=w443, length (rest)=1000 ("y")) -> (substring=w442:string)  [unwired: 1 in]
                      n187 = local write "log"(w442) -> ()
                    }
                  }
                  n188 = local read "开始/暂停"() -> (w437:bool)
                }
                frame "DR/R" {
                  n189 = disable-structure shown="禁用" {
                    frame Disabled {
                      n190 = flat-sequence {
                        frame #0 {
                          n191 = Format Date/Time String() -> (date/time string=w459:string)  [unwired: 3 in]
                          n192 = local read "log"() -> (w454:string)
                          n193 = Concatenate Strings(w459, "\t", "DR/R" ("字符串"), "\r", w454) -> (w456:string)
                          n194 = String Subset(string=w456, length (rest)=1000 ("y")) -> (substring=w455:string)  [unwired: 1 in]
                          n195 = local write "log"(w455) -> ()
                        }
                      }
                    }
                    frame Enabled {
                    }
                  }
                  n196 = disable-structure shown="禁用" {
                    disable-tunnel: w449 -> [w464 _]
                    disable-tunnel: w448 -> [w463 _]
                    frame Disabled {
                      n197 = local read item#-1() -> (w460)
                      n198 = Index Array(array=w460, index=w464) -> (element=w461)
                      n199 = call "dR.vi"() -> ("Image Dst Out"=w462:T1)  [unwired: 11 in]
                      n200 = case shown="0" w463 {
                        selector: w463 -> [_ w469]
                        tunnel: w462 -> [w466 w470]
                        tunnel: w461 -> [w465 w472]
                        frame 0 {
                          n201 = call "IMAQ Copy"("Image Dst"=w465, "Image Src"=w466) -> ()  [unwired: 4 in, 2 out]
                        }
                        frame 1, Default {
                          n202 = Increment(x=w469) -> (x+1=w468:i32)
                          n203 = call "IMAQ Multiply"("Image Src A"=w472, "Constant"=w469, "Image Dst"=w472) -> ("Image Dst Out"=w471:T1)  [unwired: 4 in, 1 out]
                          n204 = call "IMAQ Add"("Image Src A"=w471, "Image Dst"=w471, "Image Src B"=w470) -> ("Image Dst Out"=w467:T1)  [unwired: 4 in, 1 out]
                          n205 = call "IMAQ Divide"("Image Src A"=w467, "Constant"=w468, "Image Dst"=w467) -> ()  [unwired: 4 in, 2 out]
                        }
                      }
                    }
                    frame Enabled {
                    }
                  }
                  n206 = local read "开始/暂停"() -> (w450:bool)
                }
                frame "wait heart" {
                  n207 = flat-sequence {
                    frame #0 {
                      n208 = Format Date/Time String() -> (date/time string=w482:string)  [unwired: 3 in]
                      n209 = local read "log"() -> (w477:string)
                      n210 = Concatenate Strings(w482, "\t", "wait heart" ("字符串"), "\r", w477) -> (w479:string)
                      n211 = String Subset(string=w479, length (rest)=1000 ("y")) -> (substring=w478:string)  [unwired: 1 in]
                      n212 = local write "log"(w478) -> ()
                    }
                  }
                  n213 = local read "开始/暂停"() -> (w474:bool)
                }
                frame "wait calibrate" {
                  n214 = local read "开始/暂停"() -> (w484:bool)
                }
                frame "openLightShutter" {
                  n215 = flat-sequence {
                    frame #0 {
                      n216 = local read "address"() -> (w495:i16)
                      n217 = call "Write_para_port2_singalChange.vi"("索引"=1, "布尔"=TRUE, "address"=w495) -> ()  [unwired: 8 in, 1 out]
                    }
                  }
                  n218 = flat-sequence {
                    frame #0 {
                      n219 = Format Date/Time String() -> (date/time string=w494:string)  [unwired: 3 in]
                      n220 = local read "log"() -> (w489:string)
                      n221 = Concatenate Strings(w494, "\t", "open light shutter" ("字符串"), "\r", w489) -> (w491:string)
                      n222 = String Subset(string=w491, length (rest)=1000 ("y")) -> (substring=w490:string)  [unwired: 1 in]
                      n223 = local write "log"(w490) -> ()
                    }
                  }
                  n224 = local read "开始/暂停"() -> (w486:bool)
                }
                frame "closeLightShutter" {
                  n225 = flat-sequence {
                    frame #0 {
                      n226 = local read "address"() -> (w508:i16)
                      n227 = call "Write_para_port2_singalChange.vi"("索引"=1, "布尔"=FALSE, "address"=w508) -> ()  [unwired: 8 in, 1 out]
                    }
                  }
                  n228 = flat-sequence {
                    frame #0 {
                      n229 = Format Date/Time String() -> (date/time string=w507:string)  [unwired: 3 in]
                      n230 = local read "log"() -> (w502:string)
                      n231 = Concatenate Strings(w507, "\t", "close light shutter" ("字符串"), "\r", w502) -> (w504:string)
                      n232 = String Subset(string=w504, length (rest)=1000 ("y")) -> (substring=w503:string)  [unwired: 1 in]
                      n233 = local write "log"(w503) -> ()
                    }
                  }
                  n234 = local read "开始/暂停"() -> (w499:bool)
                }
                frame "writing data" {
                  n235 = while {
                    stop <- w521 continue-if-true
                    n236 = local read "writeing data"() -> (w521:bool)
                    n237 = Wait (ms)(milliseconds to wait=u32 1 ("等待时间（毫秒）")) -> ()  [unwired: 1 out]
                  }
                  n238 = flat-sequence {
                    frame #0 {
                      n239 = Format Date/Time String() -> (date/time string=w520:string)  [unwired: 3 in]
                      n240 = local read "log"() -> (w515:string)
                      n241 = Concatenate Strings(w520, "\t", "writing data" ("字符串"), "\r", w515) -> (w517:string)
                      n242 = String Subset(string=w517, length (rest)=1000 ("y")) -> (substring=w516:string)  [unwired: 1 in]
                      n243 = local write "log"(w516) -> ()
                    }
                  }
                  n244 = local read "开始/暂停"() -> (w512:bool)
                }
              }
            }
            "Stim_ID" <- w332
          }
          n245 = Flush File(refnum=w265) -> (refnum out=w264:refnum<file>)  [unwired: 1 in, 1 out]
          n246 = flat-sequence {
            tunnel: "Pra_DR/R parameter" -> [w295]
            tunnel: w264 -> [w294]
            tunnel: w266 -> [w293]
            frame #0 {
              n247 = local read "Pra_stim ID"() -> (w292:u8[])
              n248 = call "dR_R_ForFile.vi"("DR/R parameter"=w295, "clip ratio"="Pra_clip ratio", "stim ID"=w292, "OnlineMap"="Pra_OnlineMap", "blkIndex"=w293, "BlkFile"=w294) -> ("onLineMapOutput"=w290:T1[])  [unwired: 5 in]
              "onLineMapOutput" <- w290
              n249 = Format Date/Time String() -> (date/time string=w289:string)  [unwired: 3 in]
              n250 = local read "log"() -> (w284:string)
              n251 = call "IMAQ Browser Setup"("Image Ratio"=sgl 1.0, "Browser Info"=T16 {"Browser Size"={"X"=1200, "Y"=256}, "Images per Line"=6, "Background Color"=10066329, "Frame Size"=3, "Frame Style"=enum."Raised"}, "Image In"="browse" ("Image Name")) -> ("Image Browser Out"=w275:T1)  [unwired: 1 in, 3 out]
              n252 = local read "FrameHeight"() -> (w280:i64)
              n253 = local read "FrameWidth"() -> (w281:i64)
              n254 = Concatenate Strings(w289, "\t", "On Line Map" ("字符串"), "\r", w284) -> (w286:string)
              n255 = call "IMAQ Browser Focus Setup"("Focus Color"=u32 16711680, "Image Browser In"=w275) -> ("error out"=w271:errorcluster, "Image Browser Out"=w274:T1)  [unwired: 2 in]
              n256 = String Subset(string=w286, length (rest)=1000 ("y")) -> (substring=w285:string)  [unwired: 1 in]
              n257 = for {
                N: 16 -> [_]
                tunnel: w290 -> [w302] mode=indexing
                tunnel: w281 -> [_]
                tunnel: w280 -> [_]
                tunnel: w274 -> [w307]
                tunnel: w271 -> [_]
                i -> [w308]
                w299 = 3 items=["White", "Black", "Inverted", "Black on White", "White on Black"] ("Color")
                (unwired) u32 13816530 ("BG Color (Transparent)")
                w304 = T4 4 items=["Grayscale (U8)", "Grayscale (I16)", "Grayscale (SGL)", "Complex (CSG)", "RGB (U32)", "HSL (U32)", "RGB (U64)", "Grayscale (U16)"] ("Image Type")
                w310 = "write file data" ("替换字符串(\"\")")
                w313 = T4 0 items=["Grayscale (U8)", "Grayscale (I16)", "Grayscale (SGL)", "Complex (CSG)", "RGB (U32)", "HSL (U32)", "RGB (U64)", "Grayscale (U16)"] ("Image Type")
                n258 = call "IMAQ GetImageInfo"("Image"=w302) -> ("Image Name"=w298:string)  [unwired: 3 in, 7 out]
                n259 = call "IMAQ Cast Image"("Image Type"=w304, "Image Dst"="browseTemp" ("Image Name"), "Image Src"=w302) -> ("Image Dst Out"=w301:T1)  [unwired: 7 in, 1 out]
                n260 = call "IMAQ GetImageInfo"("Image"=w310) -> ("error out"=w311:errorcluster)  [unwired: 3 in, 7 out]
                n261 = case shown="错误" w311 {
                  tunnel: w310 -> [w325 w327]
                  tunnel: [w325 w326] -> w309
                  frame No Error {
                  }
                  frame Error {
                    w328 = T4 0 items=["Grayscale (U8)", "Grayscale (I16)", "Grayscale (SGL)", "Complex (CSG)", "RGB (U32)", "HSL (U32)", "RGB (U64)", "Grayscale (U16)"] ("Image Type")
                    n262 = call "IMAQ Create"("Image Name"=w327, "Image Type"=w328) -> ("New Image"=w326:T1)  [unwired: 3 in, 1 out]
                  }
                }
                n263 = call "IMAQ Draw Text"("String"=w298, "Color"=w299, "Font, Size & Style"=T17 {"Desired Font (Application)"=enum."User-specified Font", "[User-specified Font]"={"Font Name"="arial", "Size"=50, "Strikeout?"=FALSE, "Italic?"=FALSE, "Underline?"=FALSE, "Outline?"=FALSE, "Shadow?"=FALSE, "Bold?"=TRUE, "Rotation Angle"=0.0}, "Horizontal Alignment"=0, "Vertical Alignment"=1}, "Image Dst"=w301, "Image Src"=w301) -> ("Image Dst Out"=w297:T1)  [unwired: 3 in, 3 out]
                n264 = Number To Decimal String(number=w308, width (-)=i16 2 ("宽度(-)")) -> (decimal integer string=w322:string)
                n265 = call <vilib>:"Space Constant.vi"() -> ("String"=w321:string)
                n266 = local read "Pra_文件名"() -> (w324:string)
                n267 = Search and Replace String(replace all?=TRUE ("替换全部？(F)"), input string=w322, search string=w321, replace string="0" ("替换字符串(\"\")")) -> (result string=w317:string)  [unwired: 4 in, 3 out]
                n268 = call "IMAQ Browser Insert"("Image Browser In"=w307, "Image to Add"=w297) -> ("Image Browser Out"=w306:T1)  [unwired: 5 in, 4 out]
                n269 = call "IMAQ WindDraw"("Window Number (0...15)"=0, "Image"=w306) -> ()  [unwired: 8 in, 2 out]
                n270 = local read "Pra_Blk目录"() -> (w312:path)
                n271 = Concatenate Strings(w324, "_" ("字符串"), w317, ".bmp" ("字符串")) -> (w315:string)
                n272 = call "IMAQ Cast Image"("Image Type"=w313, "Image Dst"=w309, "Image Src"=w302) -> ("Image Dst Out"=w305:T1)  [unwired: 7 in, 1 out]
                n273 = Build Path(base path=w312, name or relative path=w315) -> (appended path=w314:path)
                n274 = call-poly "IMAQ Write File 2"("File Path"=w314, "Image"=w305) -> ()  [unwired: 8 in, 2 out]
              }
              n275 = local write "log"(w285) -> ()
            }
          }
        }
        frame Error {
          n276 = local write "开始/暂停"(TRUE ("开始/暂停")) -> ()
          n277 = One Button Dialog(message="blk exist, please change the file name" ("消息")) -> ()  [unwired: 1 in, 1 out]
        }
      }
      "block" <- w249
    }
    n278 = Array Size(array="Pra_stim ID") -> (size(s)=w217:i32)
    n279 = local write "Stimuli"(w217) -> ()
    n280 = property on="Pra_bin" class="Enum (严格)"("DisabledEnum"=w214) -> ()  [unwired: 2 in, 2 out]
    n281 = property on="SaveParameter" class="Bool"("DisabledEnum"=w214) -> ()  [unwired: 2 in, 2 out]
    n282 = property on="Pra_binType" class="Enum (严格)"("DisabledEnum"=w214) -> ()  [unwired: 2 in, 2 out]
    n283 = local read "停止循环"() -> (w223:bool)
    n284 = node-c288() -> ()  [unwired: 1 in, 1 out]
  }
  n285 = call "IMAQ Create"("Image Name"="ScreenSensor", "Image Type"=w6) -> ("New Image"=w5:T1)  [unwired: 3 in, 1 out]
  n286 = node-c288() -> (w9:T10)  [unwired: 4 in]
  n287 = node-c288(535 ("优先级")) -> (w73:T10)  [unwired: 3 in]
  n288 = timed-loop {
    timing: w9 -> [_]
    timing-out: [_] -> w8
    stop <- FALSE stop-if-true
    # "this step will return true if pallel port doesn't connect any signal.That means this loop only run once."
    n289 = node-c288() -> ()  [unwired: 1 in, 1 out]
    n290 = local read "address"() -> (w528:i16)
    n291 = call "read_para_port1.vi"("address"=w528) -> ("port1（5元素）"=w530:bool[])  [unwired: 9 in, 1 out]
    n292 = Index Array(array=w530, index=3 ("索引")) -> (element=→"ScreenSensor":bool)
    n293 = node-c288() -> ()  [unwired: 1 in, 1 out]
  }
  n294 = timed-loop {
    tunnel: [w544] -> w68
    tunnel: [w582] -> w17
    tunnel: w25 -> [w561]
    tunnel: w13 -> [w581]
    tunnel: w14 -> [w580]
    tunnel: [w579] -> w53
    timing: w73 -> [_]
    timing-out: [_] -> w72
    tunnel: w49 -> [w570]
    tunnel: w21 -> [w565]
    tunnel: w44 -> [w575]
    tunnel: w40 -> [_]
    tunnel: w41 -> [w574]
    tunnel: w38 -> [w573]
    shift-right: [w568] -> _
    shift-left: 1 -> [w569]
    shift-right: [w567] -> _
    shift-left: w33 -> [w566]
    tunnel: w30 -> [w563]
    tunnel: w29 -> [w562]
    tunnel: w28 -> [w559]
    tunnel: w27 -> [w558]
    tunnel: "Pra_binType" -> [w557]
    shift-right: [w551] -> _
    shift-left: _ -> [w555]
    shift-right: [w552] -> _
    shift-left: _ -> [w550]
    tunnel: w22 -> [w549]
    shift-right: [w548] -> _
    shift-left: _ -> [w547]
    tunnel: [w546] -> w10
    tunnel: w5 -> [w533]
    i -> [w553]
    stop <- w576 stop-if-true
    w542 = u16 1 items=["Line", "Rectangle", "Oval"] ("Shape to draw")
    w543 = u16 1 items=["Frame", "Paint", "Invert Frame", "Invert Paint"] ("Draw Mode")
    n295 = node-c288() -> (→"循环持续时间":i64)  [unwired: 1 in]
    n296 = flat-sequence {
      frame #0 {
      }
      frame #1 {
        n297 = event shown="[3] \"LoadParameter\": 值改变" {
          selector: _ -> [_ _ _ _]
          dyn-events: _ -> [_ _ _ _]
          timeout: 0 -> [_ _ _ _]
          event Timeout {
            n298 = event-data() -> ()  [unwired: 1 in, 2 out]
          }
          event "停止": Value Change {
            n299 = event-data() -> ("NewVal"=w673:bool)  [unwired: 1 in, 1 out]
            n300 = case shown="真" w673 {
              selector: w673 -> [_ w675]
              tunnel: [FALSE w675] -> _
              frame False {
              }
              frame True {
                n301 = local write "开始/暂停"(w675) -> ()
                "停止循环" <- w675
              }
            }
          }
          event "SaveParameter": Value Change {
            n302 = event-data() -> ()  [unwired: 1 in, 1 out]
            n303 = call "文件对话框"("prompt"="SaveParameterTo", "pattern (all files)"="*.prmf", "pattern label"="Flowbit") -> ("selected path"=w677:path, "error out"=w679:errorcluster)  [unwired: 9 in, 2 out]
            n304 = case shown="无错误" w679 {
              tunnel: w677 -> [w682 _]
              frame No Error {
                n305 = control-ref of="本VI"() -> (w686:refnum<vi>)
                n306 = invoke class="VI" method="Ctrl Val.Get All"(reference=w686, "Controls"=TRUE ("输入控件")) -> ("Get All Control Values Variant"=w685:cluster{"Name":string, "Variant Data":variant}[])  [unwired: 2 in, 3 out]
                n307 = for {
                  tunnel: w685 -> [w690] mode=indexing
                  shift-right: [w689] -> w683
                  shift-left: cluster{"Name":string, "Variant Data":variant}[] [] -> [w688]
                  i -> [w687]
                  n308 = Unbundle By Name(w690) -> ("Name"=w695:string)
                  n309 = String Subset(string=w695, length (rest)=4 ("长度（剩余）")) -> (substring=w693:string)  [unwired: 1 in]
                  n310 = Equal?(x=w693, y="Pra_") -> (x = y?=w691:bool)
                  n311 = case shown="真" w691 {
                    tunnel: w690 -> [_ w700]
                    tunnel: [w696 w699] -> w689
                    tunnel: w688 -> [w696 w698]
                    tunnel: w687 -> [_ w697]
                    frame False {
                    }
                    frame True {
                      n312 = case shown="0" w697 {
                        tunnel: w700 -> [w702 w705]
                        tunnel: [w701 w704] -> w699
                        tunnel: w698 -> [_ w703]
                        frame 0 {
                          n313 = Build Array(w702) -> (w701:cluster{"Name":string, "Variant Data":variant}[])
                        }
                        frame 1, Default {
                          n314 = Build Array (concatenate)(w703, w705) -> (w704:cluster{"Name":string, "Variant Data":variant}[])
                        }
                      }
                    }
                  }
                }
                n315 = Write to Binary File(file (use dialog)=w682, data=w683) -> ()  [unwired: 4 in, 3 out]
              }
              frame Error {
              }
            }
          }
          event "LoadParameter": Value Change {
            n316 = event-data() -> ()  [unwired: 1 in, 1 out]
            n317 = call "文件对话框2"("prompt"="LoadParameter", "pattern (all files)"="*.prmf", "pattern label"="Flowbit") -> ("selected path"=w706:path, "error out"=w707:errorcluster)  [unwired: 9 in, 2 out]
            n318 = case shown="无错误" w707 {
              tunnel: w706 -> [w715 _]
              tunnel: [w711 _] -> _
              frame No Error {
                n319 = Read from Binary File(5:cluster{"Name":string, "Variant Data":variant}[] [], 11:w715) -> (2:w712:cluster{"Name":string, "Variant Data":variant}[])  [unwired: 4 in, 3 out]
                n320 = control-ref of="本VI"() -> (w713:refnum<vi>)
                n321 = for {
                  tunnel: w713 -> [w721]
                  tunnel: w712 -> [w720] mode=indexing
                  tunnel: [w716] -> w711 mode=indexing
                  n322 = Unbundle By Name(w720) -> ("Name"=w719:string, "Variant Data"=w718:variant)
                  n323 = invoke class="VI" method="Ctrl Val.Set"(reference=w721, "Control Name"=w719, "Value"=w718) -> (error out=w717:errorcluster)  [unwired: 2 in, 4 out]
                  n324 = call <vilib>:"Clear Errors.vi"("error in (no error)"=w717) -> ("error out"=w716:errorcluster)  [unwired: 6 in]
                }
              }
              frame Error {
              }
            }
          }
        }
      }
    }
    n325 = Get Queue Status(queue=w565) -> (queue out=w564:refnum<queue>, # elements in queue=→"队列中元素数量":i32)  [unwired: 2 in, 6 out]
    n326 = local read "ScreenSensor"() -> (w541:bool)
    n327 = case shown="\"2*2\"" "Pra_bin" {
      tunnel: w563 -> [_ w657]
      tunnel: w562 -> [_ w652]
      tunnel: w561 -> [w649 w656]
      tunnel: [w649 w655] -> w534
      tunnel: w559 -> [w648 w661]
      tunnel: w558 -> [w647 w658]
      tunnel: w557 -> [_ w651]
      tunnel: [errorcluster {"status"=FALSE, "code"=0, "source"=""} ("error out") w650] -> w536
      frame "1*1", Default {
        n328 = local write "FrameHeight"(w647) -> ()
        n329 = local write "FrameWidth"(w648) -> ()
      }
      frame "2*2" {
        n330 = Divide(x=w661, y=2) -> (x/y=w654:dbl)
        n331 = Divide(x=w658, y=2) -> (x/y=w653:dbl)
        n332 = local write "FrameWidth"(w654) -> ()
        n333 = case shown="\"Extract\", 默认" w651 {
          tunnel: w657 -> [_ w670]
          tunnel: w656 -> [w664 w671]
          tunnel: [w663 w667] -> w655
          tunnel: w654 -> [_ w669]
          tunnel: w653 -> [_ w668]
          tunnel: w652 -> [_ w666]
          tunnel: [errorcluster {"status"=FALSE, "code"=0, "source"=""} ("error out") w665] -> w650
          frame "Extract", Default {
            n334 = call "Bin2.vi"("Image Src"=w664) -> ("Image"=w663:T1)  [unwired: 10 in]
          }
          frame "Resample" {
            n335 = call "IMAQ Resample"("X Resolution"=w669, "Y Resolution"=w668, "Interpolation Type"=w666, "Image Dst"=w670, "Image Src"=w671) -> ("error out"=w665:errorcluster, "Image Dst Out"=w667:T1)  [unwired: 5 in]
          }
        }
        n336 = local write "FrameHeight"(w653) -> ()
      }
    }
    n337 = Select(t=i16 4000, s=w541, f=i16 0) -> (s? t:f=w540:i16)
    n338 = call "IMAQ Draw"("Draw Mode"=w543, "Shape to draw"=w542, "Pixel Color"=w540, "error in (no error)"=w536, "Coordinates"=i32[] [0, 0, 20, 20], "Image Dst"=w533, "Image Src"=w534) -> ("error out"=w535:errorcluster, "Image Dst Out"=w544:T1)  [unwired: 3 in]
    n339 = local read "Recording"() -> (w551:bool)
    n340 = case shown="真" w551 {
      tunnel: w564 -> [w590 w604]
      tunnel: w544 -> [_ w609]
      tunnel: w570 -> [_ w608]
      tunnel: w569 -> [_ w600]
      tunnel: [1 w605] -> w568
      tunnel: w566 -> [_ w601]
      tunnel: [u32[][] [] w603] -> w567
      tunnel: [w591 w597] -> w548
      tunnel: w547 -> [_ w598]
      tunnel: [w590 w596] -> w546
      tunnel: w535 -> [_ w595]
      frame False {
        n341 = local read "Pra_FramesPerStim"() -> (w591:i64)
      }
      frame True {
        n342 = call "IMAQ Copy"("error in (no error)"=w595, "Image Dst"=w608, "Image Src"=w609) -> ("error out"=w594:errorcluster, "Image Dst Out"=w607:T1)  [unwired: 3 in]
        n343 = call "IMAQ ImageToArray"("error in (no error)"=w594, "Image"=w607) -> ("Image Pixels (I16)"=w602:i16[][])  [unwired: 2 in, 4 out]
        n344 = Greater?(x="Pra_FrameBin", y=w600) -> (0:w606:bool)
        n345 = case shown="假" w606 {
          tunnel: w600 -> [_ w630]
          tunnel: [1 w629] -> w605
          tunnel: w604 -> [w619 w627]
          tunnel: [u32[][] [] w632] -> w603
          tunnel: w602 -> [w618 w634]
          tunnel: w601 -> [w617 w633]
          tunnel: w600 -> [_ w631]
          tunnel: "Pra_FrameBin" -> [w614 _]
          tunnel: w598 -> [w613 w628]
          tunnel: [w611 w628] -> w597
          tunnel: [w610 w627] -> w596
          frame False {
            n346 = case shown="0, 默认" w614 {
              tunnel: w618 -> [w624 w626]
              tunnel: w617 -> [w623 _]
              tunnel: [w622 w625] -> w615
              frame 0, Default {
                n347 = Add(x=w624, y=w623) -> (x+y=w622:u32[][])
              }
              frame 1 {
                n348 = To Unsigned Long Integer(number=w626) -> (unsigned 32bit integer=w625:u32[][])
              }
            }
            n349 = Decrement(x=w613) -> (x-1=w611:i64)
            n350 = Less Or Equal To 0?(x=w611) -> (x <= 0?=w612:bool)
            n351 = case shown="真" w612 {
              frame False {
              }
              frame True {
                n352 = local write "Recording"(FALSE ("Recording")) -> ()
              }
            }
            n353 = Enqueue Element(queue=w619, element=w615) -> (queue out=w610:refnum<queue>)  [unwired: 2 in, 2 out]
          }
          frame True {
            n354 = case shown="1" w631 {
              tunnel: w634 -> [w635 w638]
              tunnel: w633 -> [_ w637]
              tunnel: [w635 w636] -> w632
              frame 1 {
              }
              frame 0, Default {
                n355 = Add(x=w638, y=w637) -> (x+y=w636:u32[][])
              }
            }
            n356 = Increment(x=w630) -> (x+1=w629:i32)
          }
        }
      }
    }
    n357 = Not Equal?(x=w551, y=w555) -> (x != y?=w554:bool)
    n358 = case shown="真" "热图" {
      tunnel: w575 -> [_ w731]
      tunnel: w544 -> [w722 w729]
      tunnel: [w722 w728] -> w572
      tunnel: w574 -> [_ w726]
      tunnel: w573 -> [_ w725]
      tunnel: w549 -> [_ _]
      tunnel: w535 -> [_ w723]
      frame False {
      }
      frame True {
        w727 = T4 4 items=["Grayscale (U8)", "Grayscale (I16)", "Grayscale (SGL)", "Complex (CSG)", "RGB (U32)", "HSL (U32)", "RGB (U64)", "Grayscale (U16)"] ("Image Type")
        n359 = call "IMAQ Copy"("error in (no error)"=w723, "Image Dst"=w731, "Image Src"=w729) -> ("Image Dst Out"=w730:T1)  [unwired: 3 in, 1 out]
        n360 = call "IMAQ Divide"("Image Src A"=w730, "Constant"=sgl 256.0, "Image Dst"=w730) -> ("Image Dst Out"=w724:T1)  [unwired: 4 in, 1 out]
        n361 = call "IMAQ Cast Image"("Image Type"=w727, "Lookup Table"=w725, "Image Dst"=w726, "Image Src"=w724) -> ("Image Dst Out"=w728:T1)  [unwired: 6 in, 1 out]
      }
    }
    "Image 2" <- w572
    n362 = case shown="真" w554 {
      tunnel: w553 -> [_ w640]
      tunnel: [w639 w640] -> w552
      tunnel: w550 -> [w639 w641]
      tunnel: w551 -> [_ w642]
      tunnel: w550 -> [_ _]
      frame False {
      }
      frame True {
        n363 = case shown="假" w642 {
          tunnel: w641 -> [w644 _]
          tunnel: w640 -> [w643 _]
          frame False {
            n364 = Subtract(x=w643, y=w644) -> (x-y=→"grabLoop":i32)
          }
          frame True {
          }
        }
      }
    }
    n365 = event shown="[1] \"shutter\": 值改变" {
      selector: _ -> [_ _]
      dyn-events: _ -> [_ _]
      timeout: 0 -> [_ _]
      event Timeout {
        n366 = event-data() -> ()  [unwired: 1 in, 2 out]
      }
      event "shutter": Value Change {
        n367 = event-data() -> ("NewVal"=w583:bool)  [unwired: 1 in, 4 out]
        n368 = case shown="假" w583 {
          frame False {
            n369 = flat-sequence {
              frame #0 {
                n370 = local read "address"() -> (w584:i16)
                n371 = call "Write_para_port2_singalChange.vi"("索引"=1, "布尔"=FALSE, "address"=w584) -> ()  [unwired: 8 in, 1 out]
              }
            }
          }
          frame True {
            n372 = flat-sequence {
              frame #0 {
                n373 = local read "address"() -> (w587:i16)
                n374 = call "Write_para_port2_singalChange.vi"("索引"=1, "布尔"=TRUE, "address"=w587) -> ()  [unwired: 8 in, 1 out]
              }
            }
          }
        }
      }
    }
    n375 = local read "停止循环"() -> (w576:bool)
    n376 = call <vilib>:"Wait For Frame.vi"("error in (no error)"=w581, "Timeout (mS)"=u32 5000, "RefBrdIn"=w580) -> ("error out"=w582:errorcluster, "RefBrdOut"=w579:u32)  [unwired: 7 in]
    n377 = node-c288() -> ()  [unwired: 1 in, 1 out]
  }
  n378 = node-c288(w8) -> ()  [unwired: 1 out]
  n379 = node-c288(w72) -> ()  [unwired: 1 out]
  n380 = call "IMAQ WindClose"("Close All Windows (False)"=TRUE, "error in (no error)"=w17) -> ("error out"=w16:errorcluster)  [unwired: 4 in]
  n381 = call <vilib>:"Stop.vi"("error in (no error)"=w16, "Image In"=w68, "RefBrdIn"=w53) -> ("error out"=w64:errorcluster, "Image"=w67:T1, "RefBrdOut"=w52:u32)  [unwired: 6 in]
  n382 = call <vilib>:"Cleanup.vi"("error in (no error)"=w64, "Image In"=w67, "RefBrdIn"=w52) -> ("error out"=w65:errorcluster, "Image"=w66:T1, "RefBrdOut"=w51:u32)  [unwired: 6 in]
  n383 = call <vilib>:"Close.vi"("error in (no error)"=w65, "RefBrdIn"=w51) -> ("error out"=w50:errorcluster)  [unwired: 8 in, 1 out]
  n384 = call "Imaq Dispose"("Image"=w66, "error in (no error)"=w50) -> ("error out"=w12:errorcluster)  [unwired: 4 in]
  n385 = flat-sequence {
    tunnel: w12 -> [w738]
    tunnel: [w737] -> w11
    tunnel: w10 -> [w736]
    tunnel: w11 -> [_]
    frame #0 {
      n386 = Flush Queue(queue=w736, error in (no error)=w738) -> (error out=w737:errorcluster)  [unwired: 2 out]
    }
    frame #1 {
      (unwired) 0.0 ("Output Voltage (V) (0.0)")
    }
    frame #2 {
      n387 = Stop(stop? (T)=TRUE ("停止？(T)")) -> ()
    }
  }
  n388 = node-c288(w3) -> ()  [unwired: 1 out]
